vi "Benchmark SV Receive LV2012 - NI Verified - 3.vi"() -> ()   [LabVIEW 2015]
panel:
  out "Built-In Encoder":i32[](array[numeric])
  in  "file path (dialog if empty)":path=path "D:/TFS-Labview/Usefull LabView Program/Benchmark SV  LV2012 NI Verified Folder/Benchmark SV  LV2012 NI Verified Folder/Example Tab-Delimited File.txt"
  out "data out":T1
  in  "stop":bool
  # "Overview:  Coding that exemplifies how to benchmark the communication of Shared Variables.\nRequirements: LabVIEW 2012 or compatible\nInstructions:\n1. Run this VI\n2. Watch the amount of time it takes to communicate on the \"Benchmark SV Send  LV2012 - NI Verified.vi\" \n3. Stop both VIs"
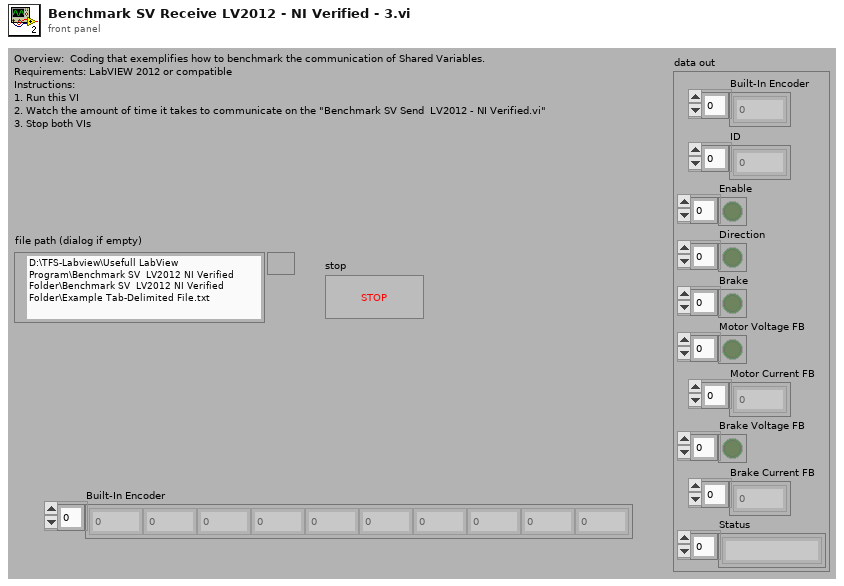
[diagram p1: front panel]
types:
  T1 = cluster{"Built-In Encoder":i32[], "ID":i16[], "Enable":bool[], "Direction":bool[], "Brake":bool[], "Motor Voltage FB":bool[], "Motor Current FB":i32[], "Brake Voltage FB":bool[], "Brake Current FB":i32[], "Status":string[]}
  T2 = enum16{"open", "replace", "create", "open or create", "replace or create", "replace or create with confirmation"}
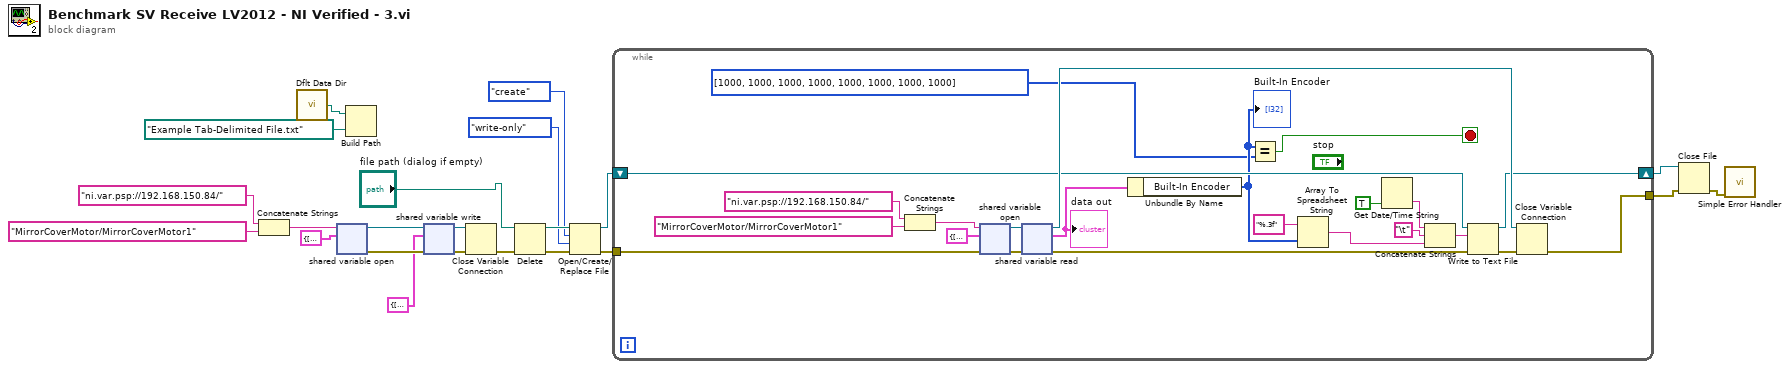
[diagram p0: block diagram]
diagram:
  n1 = Concatenate Strings("ni.var.psp://192.168.150.84/" ("string"), "MirrorCoverMotor/MirrorCoverMotor1") -> (w18:string)
  n2 = call <vilib>:"Dflt Data Dir.vi"() -> ("App:Default Data Directory"=w5:path)
  n3 = shared-variable-open(w18, T1 {"Built-In Encoder"=[], "ID"=[], "Enable"=[], "Direction"=[], "Brake"=[], "Motor Voltage FB"=[], "Motor Current FB"=[], "Brake Voltage FB"=[], "Brake Current FB"=[], "Status"=[]} ("MirrorCoverMotor")) -> (w16:refnum<k21>, w14:errorcluster)  [unwired: 2 in]
  n4 = Build Path(base path=w5, name or relative path=path "Example Tab-Delimited File.txt" ("default name")) -> ()  [unwired: 1 out]
  n5 = shared-variable-write(w16, w14, T1 {"Built-In Encoder"=[], "ID"=[], "Enable"=[], "Direction"=[], "Brake"=[], "Motor Voltage FB"=[], "Motor Current FB"=[], "Brake Voltage FB"=[], "Brake Current FB"=[], "Status"=[]} ("data in")) -> (w15:refnum<k21>, w13:errorcluster)
  n6 = Close Variable Connection(8:w13, 11:w15) -> (0:w10:errorcluster)
  n7 = Delete(path (use dialog)="file path (dialog if empty)", error in=w10) -> (deleted path=w22:path, error out=w9:errorcluster)  [unwired: 3 in, 1 out]
  n8 = Open/Create/Replace File(file path (use dialog)=w22, error in=w9, operation (0:open)=T2."create", access (0:read/write)=enum16{"read/write", "read-only", "write-only"}."write-only") -> (refnum out=w19:refnum<file>, error out=w8:errorcluster)  [unwired: 3 out]
  n9 = while {
    shift-right: [w30] -> w3
    shift-left: w19 -> [w31]
    tunnel: w8 -> [w27]
    tunnel: [w23] -> w1
    stop <- w25 stop-if-true
    n10 = Concatenate Strings("ni.var.psp://192.168.150.84/" ("string"), "MirrorCoverMotor/MirrorCoverMotor1") -> (w44:string)
    n11 = shared-variable-open(w44, w27, T1 {"Built-In Encoder"=[], "ID"=[], "Enable"=[], "Direction"=[], "Brake"=[], "Motor Voltage FB"=[], "Motor Current FB"=[], "Brake Voltage FB"=[], "Brake Current FB"=[], "Status"=[]} ("MirrorCoverMotor")) -> (w43:refnum<k21>, w42:errorcluster)  [unwired: 1 in]
    n12 = shared-variable-read(w43, w42) -> (w41:refnum<k21>, w29:errorcluster, w38:T1)  [unwired: 1 out]
    "data out" <- w38
    n13 = Unbundle By Name(w38) -> ("Built-In Encoder"=w26:i32[])
    "Built-In Encoder" <- w26
    n14 = Equal?(x=w26, y=i32[] [1000, 1000, 1000, 1000, 1000, 1000, 1000, 1000] ("Built-In Encoder")) -> (x = y?=w25:bool)
    n15 = Array To Spreadsheet String(array=w26, 3:"%.3f") -> (spreadsheet string=w32:string)  [unwired: 1 out]
    n16 = Get Date/Time String(want seconds? (F)=TRUE) -> (time string=w36:string)  [unwired: 2 in, 1 out]
    n17 = Concatenate Strings(w36, "\t" ("Tab"), w32) -> (w35:string)
    n18 = Write to Text File(file (use dialog)=w31, text=w35, error in=w29) -> (refnum out=w30:refnum<file>, error out=w28:errorcluster)  [unwired: 1 in, 1 out]
    n19 = Close Variable Connection(8:w28, 11:w41) -> (0:w23:errorcluster)
  }
  n20 = Close File(refnum=w3, error in=w1) -> (error out=w2:errorcluster)  [unwired: 1 out]
  n21 = call <vilib>:"Simple Error Handler.vi"("error in (no error)"=w2) -> ()  [unwired: 4 in, 5 out]
